vi "Track Target Y.vi"() -> (3 "Joystick Y":dbl)   [LabVIEW 2019]
uses:
  2021 Team Code/Robot Global Data.vi
  <vilib>/addons/control/pid/pid.llb/PID (DBL).vi
  <vilib>/addons/control/pid/NI_PID_pid.lvlib
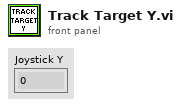
[diagram p1: front panel]
types:
  T1 = cluster{"proportional gain (Kc)":dbl, "integral time (Ti, min)":dbl, "derivative time (Td, min)":dbl}
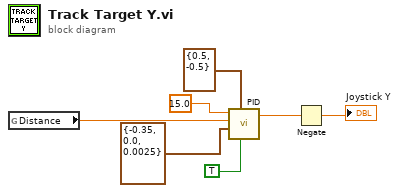
[diagram p0: block diagram]
diagram:
  n1 = global read "Robot Global Data.vi" "Distance"() -> (w4:dbl)
  n2 = call-poly <vilib>:"PID.vi"("reinitialize? (F)"=TRUE, "output range"=cluster{"output high":dbl, "output low":dbl} {"output high"=0.5, "output low"=-0.5}, "PID gains"=T1 {"proportional gain (Kc)"=-0.35, "integral time (Ti, min)"=0.0, "derivative time (Td, min)"=0.0025}, "process variable"=w4, "setpoint"=15.0) -> ("output"=w1:dbl)  [unwired: 5 in, 1 out]
  n3 = Negate(x=w1) -> (-x=→"Joystick Y":dbl)
